vi "Read TrimOTP.vi"(0 "TSM context":T1) -> (15 "error out":errorcluster)   [LabVIEW 2020]
doc: "Trims sensitivity of the DUT by adjusting the Gain and Vbias values using Trim protocol"
uses:
  <vilib>/NI_TestStand_SemiconductorModule/NI_TestStand_Semiconductor_Module.lvlibp/PinMap/General/SemiconductorModuleContext.ctl
  Common/Instrument Control/Digital/TSM/TSM SSC Digital.ctl
  <vilib>/NI_TestStand_SemiconductorModule/NI_TestStand_Semiconductor_Module.lvlibp/PinMap/Digital Pattern/PinQueryContext/DigitalPatternPinQueryContext.lvclass
  Common/Instrument Control/Digital/SSC Digital/SSC Digital.ctl
  Common/Instrument Control/DCPower/TSM/TSM SSC DCPower.ctl
  <vilib>/NI_TestStand_SemiconductorModule/NI_TestStand_Semiconductor_Module.lvlibp/PinMap/PinQueryContext/MultiplePinMultipleSessionQueryContext/MultiplePinMultipleSessionQueryContext.lvclass
  Common/Instrument Control/DCPower/SSC DCPower/SSC DCPower.ctl
  Common/Instrument Control/Shared SubVIs/TSM Pin Abstraction/TSM Pin Information.ctl
  Common/Instrument Control/Shared SubVIs/TSM Pin Abstraction/TSM Pin Type Identifier.ctl
  Common/Instrument Control/Shared SubVIs/TSM Pin Abstraction/TSM Expanded Pin Information.ctl
  Common/DUT Control/Typedefs/DUT Read Commands.ctl
  <vilib>/NI_TestStand_SemiconductorModule/NI_TestStand_Semiconductor_Module.lvlibp/PinMap/TagProvider/TSM_PublishedDataId.ctl
  354e2fd9-1388-4924-804e-e9490b2eeb0b.vi
  46ecd2fd-2f0c-4e5f-b596-d218653973fe.vi
  354e2fd9-1388-4924-804e-e9490b2eeb0b.vi/71683651-cbc5-46e0-8522-40ce4dc1e9ef.vi
  354e2fd9-1388-4924-804e-e9490b2eeb0b.vi/5048e37d-0f89-4c33-89a7-b3c71e857334.vi
  354e2fd9-1388-4924-804e-e9490b2eeb0b.vi/0bdf4848-63d7-49b9-a33f-cfc1e4c0521b.vi
  354e2fd9-1388-4924-804e-e9490b2eeb0b.vi/b8e335d8-4854-4718-8e9f-88d363955659.vi
  Common/Instrument Control/Digital/TSM/TSM SSC Digital N Pins To M Sessions.vi
  <vilib>/NI_TestStand_SemiconductorModule/NI_TestStand_Semiconductor_Module.lvlibp/PinMap/Input Data/GetInputDataDouble.vi
  Common/Instrument Control/DCPower/SSC DCPower/Source/SSC DCPower Configure Output Enabled.vi
  Common/Instrument Control/DCPower/SSC DCPower/Source/Constant Voltage/SSC DCPower Force Voltage Array Symmetric Limits.vi
  <vilib>/NI_TestStand_SemiconductorModule/NI_TestStand_Semiconductor_Module.lvlibp/PinMap/Relay Driver/ControlRelay(s).vi
  <vilib>/NI_TestStand_SemiconductorModule/NI_TestStand_Semiconductor_Module.lvlibp/PinMap/Relay Driver/ApplyRelayConfiguration.vi
  <vilib>/Utility/High Resolution Polling Wait.vi
  <vilib>/NI_TestStand_SemiconductorModule/NI_TestStand_Semiconductor_Module.lvlibp/PinMap/General/Publish/PublishDataBoolFunctionalTest.vi
  <vilib>/NI_TestStand_SemiconductorModule/NI_TestStand_Semiconductor_Module.lvlibp
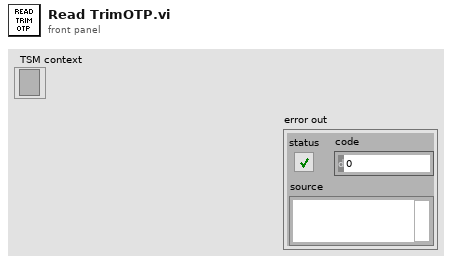
[diagram p1: front panel]
types:
  T1 = typedef "NI_TestStand_Semiconductor_Module.lvlibp/SemiconductorModuleContext.ctl" = refnum<k7>
  T2 = typedef "TSM SSC Digital.ctl" = cluster{"Pin Query Context":refnum<class "DigitalPatternPinQueryContext.lvclass">, "SSC":T3[], "Site Numbers":i32[], "Pins":tag[]}
  T3 = typedef "SSC Digital.ctl" = cluster{"Session":refnum<k15>, "Channel List":string, "Site List":string}
  T4 = typedef "TSM SSC DCPower.ctl" = cluster{"Pin Query Context":refnum<class "MultiplePinMultipleSessionQueryContext.lvclass">, "SSC":T5[], "Site Numbers":i32[], "Pins":T6[], "Pins Expanded":T8[]}
  T5 = typedef "SSC DCPower.ctl" = cluster{"Session":refnum<k15>, "Chan":string, "Channel List":string}
  T6 = typedef "TSM Pin Information.ctl" = cluster{"Pin":tag, "Type":T7, "Count":i32}
  T7 = typedef "TSM Pin Type Identifier.ctl" = enum8{"DUT Pin", "System Pin", "Pin Group", "Not Determined"}
  T8 = typedef "TSM Expanded Pin Information.ctl" = cluster{"Pin":tag, "Type":T7, "Index":i32}
  T9 = cluster{"OTP Pins":T2, "SMU_VDD_MERGED":T4, "PreTrim Sensitivity":dbl[], "PreTrimOTP":u8[], "HSD_OUT+":T2}
  T10 = typedef "NI_TestStand_Semiconductor_Module.lvlibp/TSM_PublishedDataId.ctl" = tag
  T11 = typedef "DUT Read Commands.ctl" = enum16{"Read Reg and Timeout", "Read OTP and Timeout"}
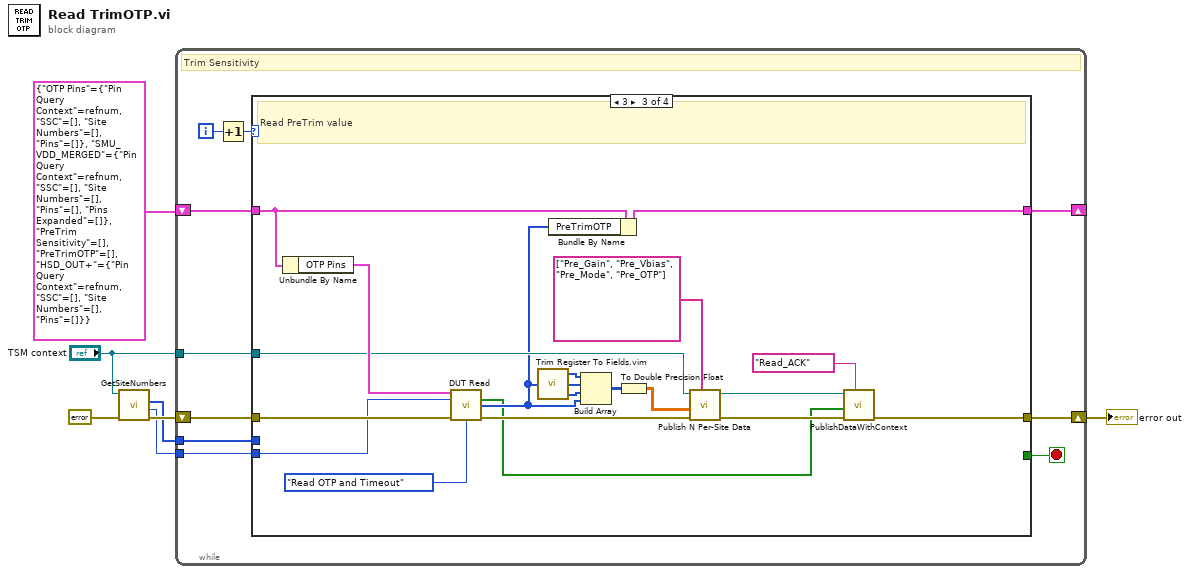
[diagram p0: block diagram]
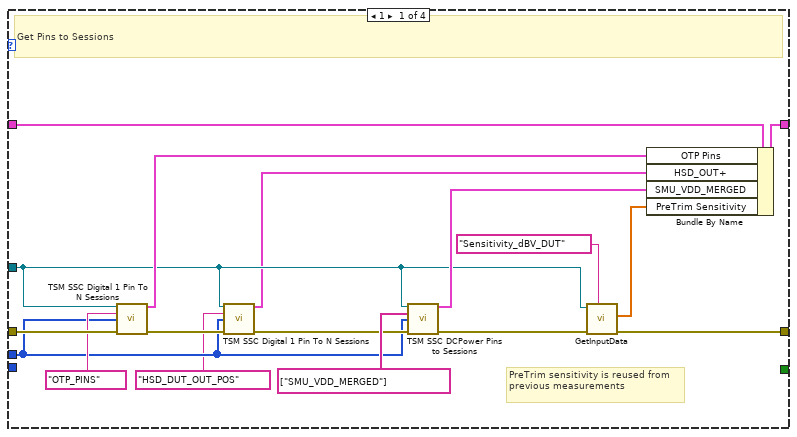
[diagram p2: hidden frame]
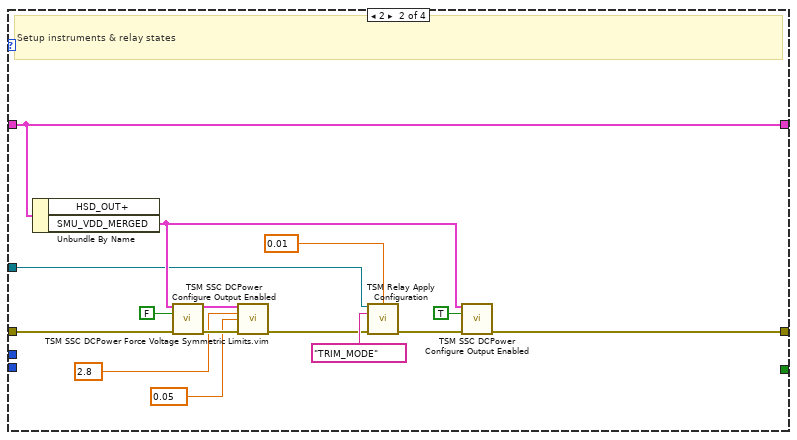
[diagram p3: hidden frame]
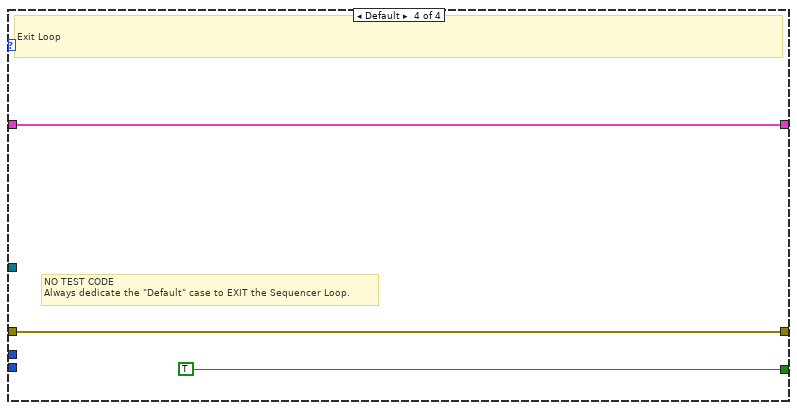
[diagram p4: hidden frame]
diagram:
  n1 = call <vilib>:"GetSiteNumbers.vi"("error in (no error)"=errorcluster {"status"=FALSE, "code"=0, "source"=""} ("error in"), "Semiconductor Module Context"="TSM context") -> ("error out"=w4:errorcluster, "Number Of Sites"=w1:i32, "Site Numbers"=w2:i32[])  [unwired: 6 in, 1 out]
  n2 = while {
    shift-right: [w15] -> w7
    shift-left: w4 -> [w16]
    tunnel: "TSM context" -> [w13]
    shift-right: [w10] -> _
    shift-left: T9 {"OTP Pins"={"Pin Query Context"=refnum, "SSC"=[], "Site Numbers"=[], "Pins"=[]}, "SMU_VDD_MERGED"={"Pin Query Context"=refnum, "SSC"=[], "Site Numbers"=[], "Pins"=[], "Pins Expanded"=[]}, "PreTrim Sensitivity"=[], "PreTrimOTP"=[], "HSD_OUT+"={"Pin Query Context"=refnum, "SSC"=[], "Site Numbers"=[], "Pins"=[]}} -> [w11]
    tunnel: w2 -> [w9]
    tunnel: w1 -> [w8]
    i -> [w17]
    stop <- w12 stop-if-true
    # "Trim Sensitivity"
    n3 = Increment(x=w17) -> (x+1=w14:i32)
    n4 = case shown="3" w14 {
      tunnel: [w26 w47 w53 w71] -> w15
      tunnel: w16 -> [w34 w49 w68 w71]
      tunnel: w13 -> [w22 w37 w58 _]
      tunnel: [_ _ _ TRUE] -> w12
      tunnel: w11 -> [w33 w45 w66 w70]
      tunnel: [w31 w45 w56 w70] -> w10
      tunnel: w9 -> [w20 _ _ _]
      tunnel: w8 -> [_ _ w67 _]
      frame 1 {
        # "PreTrim sensitivity is reused from previous measurements"
        # "Get Pins to Sessions"
        n5 = call "TSM SSC Digital 1 Pin To N Sessions.vi"("TSM context"=w22, "Pin"=tag "OTP_PINS", "Site Numbers"=w20, "error in"=w34) -> ("Digital TSM Out"=w30:T2, "error out"=w23:errorcluster)  [unwired: 10 in]
        n6 = call "TSM SSC Digital 1 Pin To N Sessions.vi"("TSM context"=w22, "Pin"=tag "HSD_DUT_OUT_POS", "Site Numbers"=w20, "error in"=w23) -> ("Digital TSM Out"=w18:T2, "error out"=w21:errorcluster)  [unwired: 10 in]
        n7 = call "TSM SSC DCPower Pins to Sessions.vi"("TSM context"=w22, "Pins"=tag[] ["SMU_VDD_MERGED"], "Site Numbers"=w20, "error in"=w21) -> ("DCPower TSM Out"=w28:T4, "error out"=w25:errorcluster)  [unwired: 10 in]
        n8 = call-poly <vilib>:"GetInputData.vi"("Input Data Id"=tag "Sensitivity_dBV_DUT", "error in (no error)"=w25, "Semiconductor Module Context"=w22) -> ("error out"=w26:errorcluster, "Data Out"=w24:dbl[])  [unwired: 6 in, 1 out]
        n9 = Bundle By Name(cluster=w33, "OTP Pins"=w30, "HSD_OUT+"=w18, "SMU_VDD_MERGED"=w28, "PreTrim Sensitivity"=w24) -> (w31:T9)
      }
      frame 2 {
        # "Setup instruments & relay states"
        n10 = Unbundle By Name(w45) -> ("SMU_VDD_MERGED"=w41:T4)  [unwired: 1 out]
        n11 = call "TSM SSC DCPower Configure Output Enabled.vi"("DCPower TSM in"=w41, "Output Enabled"=FALSE, "error in"=w49) -> ("DCPower TSM out"=w44:T4, "error out"=w48:errorcluster)  [unwired: 11 in]
        n12 = call "TSM SSC DCPower Force Voltage Symmetric Limits.vim"("DCPower TSM in"=w44, "Voltage Level (V)"=2.8, "Current Limit (A)"=0.05, "error in"=w48) -> ("error out"=w38:errorcluster)  [unwired: 10 in, 1 out]
        n13 = call "TSM Relay Apply Configuration.vi"("TSM Context"=w37, "Settling Time (0s)"=0.01, "Relay Configuration"=tag "TRIM_MODE", "error in (no error)"=w38) -> ("error out"=w40:errorcluster)  [unwired: 11 in]
        n14 = call "TSM SSC DCPower Configure Output Enabled.vi"("DCPower TSM in"=w41, "Output Enabled"=TRUE, "error in"=w40) -> ("error out"=w47:errorcluster)  [unwired: 11 in, 1 out]
      }
      frame 3 {
        # "Read PreTrim value"
        n15 = Unbundle By Name(w66) -> ("OTP Pins"=w65:T2)
        n16 = call "DUT Read.vi"("Digital TSM In"=w65, "Number Of Sites"=w67, "error in (no error)"=w68, "Operation"=DUT_Read_Commands."Read OTP and Timeout") -> ("Per-Site Pass"=w51:bool[], "Per Site Read Data"=w55:u8[], "error out"=w59:errorcluster)  [unwired: 8 in, 1 out]
        n17 = call "Trim Register To Fields.vim"("ROUT"=w55) -> ("Mode"=w62:u8[], "Vbias"=w63:u8[], "Gain"=w64:u8[])  [unwired: 2 in]
        n18 = Bundle By Name(cluster=w66, "PreTrimOTP"=w55) -> (w56:T9)
        n19 = Build Array(w64, w63, w62, w55) -> (w61:u8[][])
        n20 = To Double Precision Float(number=w61) -> (double precision float=w57:dbl[][])
        n21 = call "Publish N Per-Site Data.vi"("Published Data Id"=tag[] ["Pre_Gain", "Pre_Vbias", "Pre_Mode", "Pre_OTP"], "error in (no error)"=w59, "Data In"=w57, "Semiconductor Module Context"=w58) -> ("error out"=w54:errorcluster, "Semiconductor Module Context Out"=w52:T1)  [unwired: 6 in]
        n22 = call-poly <vilib>:"PublishDataWithContext.vi"("Published Data Id"=T10 "Read_ACK", "error in (no error)"=w54, "Data In"=w51, "Semiconductor Module Context"=w52) -> ("error out"=w53:errorcluster)  [unwired: 6 in, 1 out]
      }
      frame Default {
        # "NO TEST CODE\nAlways dedicate the \"Default\" case to EXIT the Sequencer Loop."
        # "Exit Loop"
      }
    }
  }
  "error out" <- w7
